vi "Get IPS State.vi"(0 "VISA session":refnum<visa-resource-name>="GPIB0::22::INSTR") -> (1 "State":T1(ring), 3 "dup VISA session":refnum<visa-resource-name>, 4 "Switch Heater":bool, 5 "Switch heater \nconfirmed":bool, 6 "Switch Heater Error":bool)   [LabVIEW 2019]
panel:
  out "Mode":i32
  out "SwHeater":i32
  out "Loc/Rem":i32
  out "Activity":i32
  out "SysStatus1":i32
  out "SysStatus0":i32
  out "String Read":string
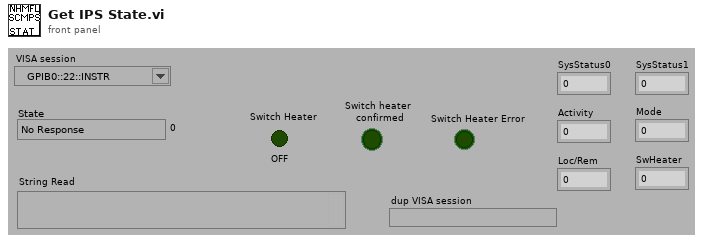
[diagram p1: front panel]
types:
  T1 = enum16{"No Response", "Ramping to programmed field ", "Holding at programmed field", "Paused", "Ramp Manual Up", "Ramp Manual Down", "Ramping to Zero", "QUENCH", "Heating Persistence Switch", "At Zero Current"}
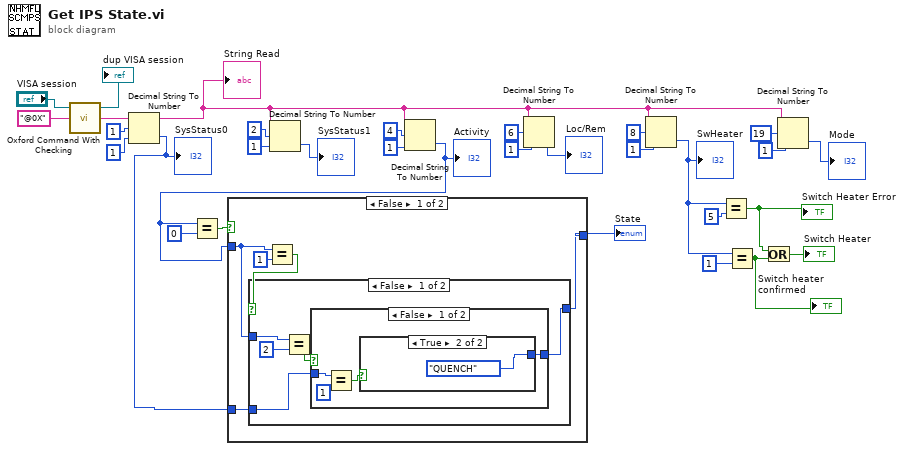
[diagram p0: block diagram]
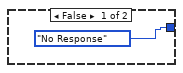
[diagram p2: hidden frame]
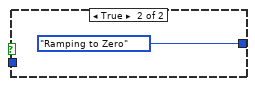
[diagram p3: hidden frame]
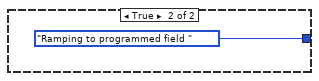
[diagram p4: hidden frame]
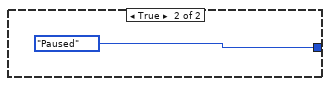
[diagram p5: hidden frame]
diagram:
  n1 = call "Oxford Command With Checking.vi"("Command"="@0X" ("Command String"), "VISA session"="VISA session") -> ("String Read"=w1:string, "dup VISA session"=→"dup VISA session":refnum<visa-resource-name>)  [unwired: 1 in, 1 out]
  "String Read" <- w1
  n2 = Decimal String To Number(string=w1, offset=1 ("offset (0)"), default (0L)=1 ("length (rest)")) -> (number=w4:i32)  [unwired: 1 out]
  "SysStatus0" <- w4
  n3 = Decimal String To Number(string=w1, offset=2, default (0L)=1 ("default (0 I32)")) -> (number=→"SysStatus1":i32)  [unwired: 1 out]
  n4 = Decimal String To Number(string=w1, offset=4, default (0L)=1 ("default (0 I32)")) -> (number=w5:i32)  [unwired: 1 out]
  "Activity" <- w5
  n5 = Equal?(x=w5, y=0) -> (x = y?=w7:bool)
  n6 = case shown="False" w7 {
    tunnel: [w33 T1."Paused" ("State")] -> w6
    tunnel: w5 -> [w32 _]
    tunnel: w4 -> [w31 _]
    frame False {
      n7 = Equal?(x=w32, y=1) -> (x = y?=w34:bool)
      n8 = case shown="False" w34 {
        tunnel: [w37 T1."Ramping to programmed field " ("State")] -> w33
        tunnel: w32 -> [w39 _]
        tunnel: w31 -> [w36 _]
        frame False {
          n9 = Equal?(x=w39, y=2) -> (x = y?=w38:bool)
          n10 = case shown="False" w38 {
            tunnel: [w41 T1."Ramping to Zero" ("State")] -> w37
            tunnel: w36 -> [w44 _]
            frame False {
              n11 = Equal?(x=w44, y=1) -> (x = y?=w42:bool)
              n12 = case shown="True" w42 {
                tunnel: [T1."No Response" ("State") T1."QUENCH" ("State")] -> w41
                frame False {
                }
                frame True {
                }
              }
            }
            frame True {
            }
          }
        }
        frame True {
        }
      }
    }
    frame True {
    }
  }
  "State" <- w6
  n13 = Decimal String To Number(string=w1, offset=6, default (0L)=1 ("default (0 I32)")) -> (number=→"Loc/Rem":i32)  [unwired: 1 out]
  n14 = Decimal String To Number(string=w1, offset=8, default (0L)=1 ("default (0 I32)")) -> (number=w10:i32)  [unwired: 1 out]
  "SwHeater" <- w10
  n15 = Equal?(x=w10, y=5) -> (x = y?=w9:bool)
  "Switch Heater Error" <- w9
  n16 = Equal?(x=w10, y=1) -> (x = y?=w3:bool)
  "Switch heater \nconfirmed" <- w3
  n17 = Or(x=w9, y=w3) -> (x .or. y?=→"Switch Heater":bool)
  n18 = Decimal String To Number(string=w1, offset=19, default (0L)=1 ("default (0 I32)")) -> (number=→"Mode":i32)  [unwired: 1 out]
